vi "ABR-Next Data File.vi"(0 "State in":T1, 7 "CAP or ABR":enum16{"CAP", "ABR"}(ring)) -> (4 "State out":T1, 6 "Run":i32, 8 "appended path":path, 15 "error out":errorcluster)   [LabVIEW 2020]
uses:
  CFTS VIs/CFTS-Experiment State.ctl
  epl-vi-lib/Utility VIs/File IO VIs/Configuration File Wrapper VIs/Config-Read Key (string).vi
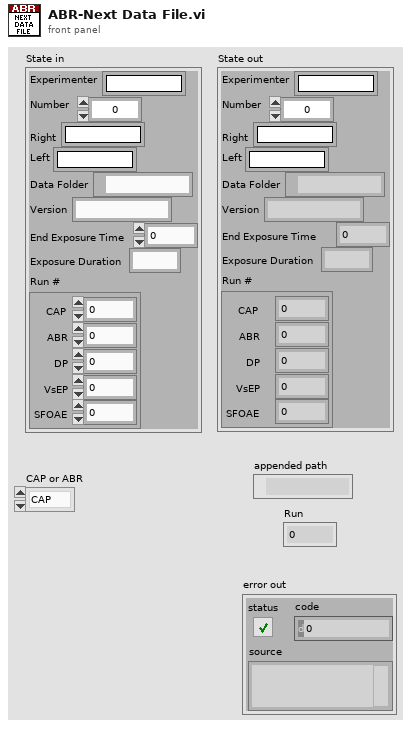
[diagram p1: front panel]
types:
  T1 = typedef "CFTS-Experiment State.ctl" = cluster{"Experimenter":string, "Number":u32, "Right":string, "Left":string, "Data Folder":path, "Version":string, "End Exposure Time":dbl, "Exposure Duration":string, "Run #":cluster{"CAP":i32, "ABR":i32, "DP":i32, "VsEP":i32, "SFOAE":i32}}
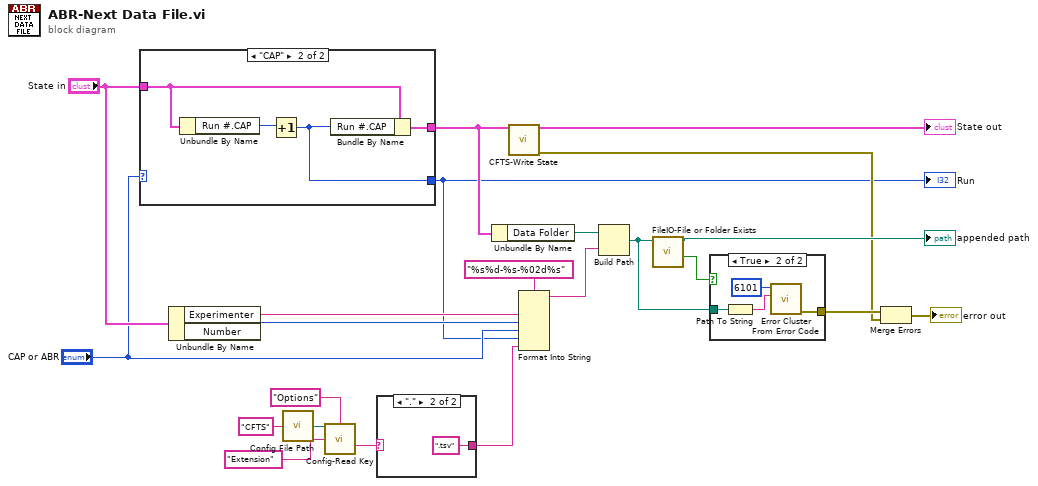
[diagram p0: block diagram]
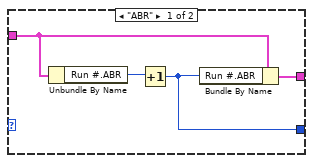
[diagram p4: hidden frame]
diagram:
  n1 = case shown="\"CAP\"" "CAP or ABR" {
    tunnel: [w26 w30] -> w16
    tunnel: [w25 w29] -> w7
    tunnel: "State in" -> [w24 w28]
    frame "ABR" {
      n2 = Unbundle By Name(w24) -> ("Run #.ABR"=w23:i32)
      n3 = Increment(x=w23) -> (x+1=w25:i32)
      n4 = Bundle By Name(cluster=w24, "Run #.ABR"=w25) -> (w26:T1)
    }
    frame "CAP" {
      n5 = Unbundle By Name(w28) -> ("Run #.CAP"=w27:i32)
      n6 = Increment(x=w27) -> (x+1=w29:i32)
      n7 = Bundle By Name(cluster=w28, "Run #.CAP"=w29) -> (w30:T1)
    }
  }
  "Run" <- w7
  n8 = Unbundle By Name("State in") -> ("Experimenter"=w10:string, "Number"=w9:u32)
  n9 = call "Config File Path.vi"("AppName"="CFTS") -> ("Default config file name"=w5:path)
  n10 = call-poly "Config-Read Key.vi"("configuration file path"=w5, "section"="Options", "key"="Extension" ("string")) -> ("value"=w2:string)  [unwired: 9 in, 3 out]
  n11 = case shown="\".\"" w2 {
    selector: w2 -> [w31 _]
    tunnel: [w31 ".tsv"] -> w1
    frame Default {
    }
    frame "." {
    }
  }
  n12 = Unbundle By Name(w16) -> ("Data Folder"=w20:path)
  n13 = call "CFTS-Write State.vi"("State"=w16) -> ("State thru"=→"State out":T1, "error out"=w14:errorcluster)  [unwired: 13 in]
  n14 = Format Into String(format string="%s%d-%s-%02d%s", w10, w9, "CAP or ABR", w7, w1) -> (resulting string=w21:string)  [unwired: 2 in, 1 out]
  n15 = Build Path(base path=w20, name or relative path=w21) -> (appended path=w13:path)
  n16 = call "FileIO-File or Folder Exists.vi"("path"=w13) -> ("Exists?"=w18:bool, "dup path"=→"appended path":path)  [unwired: 7 in, 2 out]
  n17 = case shown="True" w18 {
    tunnel: [_ w36] -> w17
    tunnel: w13 -> [_ w33]
    frame False {
    }
    frame True {
      n18 = Path To String(path=w33) -> (string=w34:string)
      n19 = call <vilib>:"Error Cluster From Error Code.vi"("error message (\"\")"=w34, "error code (0)"=6101) -> ("error out"=w36:errorcluster)  [unwired: 7 in]
    }
  }
  n20 = Merge Errors(w17, w14) -> (→"error out":errorcluster)
